vi "PH_gentec_M-Link.set Range.vi"(0 "i ref in":refnum<vi>, 2 "VISA resource in":refnum<visa-resource-name>, 5 "error in":errorcluster) -> (11 "Timeout":bool, 13 "Data read":string[](array[string]), 14 "i ref out":refnum<vi>, 16 "VISA resource out":refnum<visa-resource-name>, 17 "Error":bool, 18 "Failure":bool, 19 "error out":errorcluster)   [LabVIEW 2014, in "PH_gentec_M-Link.lvlib"]
doc: "This VI writes wanted Settings to the Device and checks the result."
uses:
  PH_gentec_M-Link.lvlib
  instr.lib/Gentec-M-Link/Driver/Type Defs/gentec-M-Link.Range Queries.ctl
  instr.lib/Gentec-M-Link/gentec-M-Link - Driver.lvlib
  PH_Basics/PH_Powermeter_BaseClass/PH_Powermeter_BaseClass.lvlib
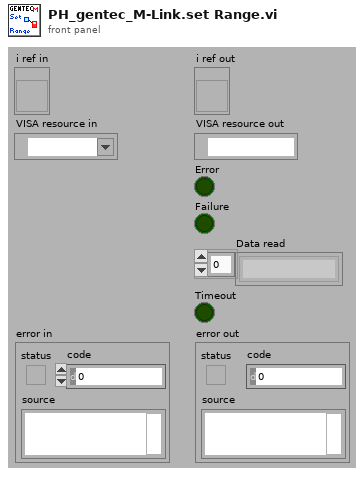
[diagram p1: front panel]
types:
  T1 = typedef "PH_Powermeter_BaseClass.lvlib/PH_Powermeter_BaseClass.i attribute.ctl" = cluster{"GUI References":T2, "Connection":T3, "Head Attributes":T5, "VISA resource":refnum<visa-resource-name>, "Energy":T6, "Service ID Energy":i32, "Wanted Settings":T7, "Current Settings":T7}
  T2 = typedef "PH_Powermeter_BaseClass.lvlib/PH_Powermeter_BaseClass.GUI Refs.ctl" = cluster{"Head Attributes":refnum<vi>, "Energy":refnum<vi>, "Connection":refnum<vi>, "VISA Resource":refnum<vi>, "Scaling Factor":refnum<vi>, "Range":refnum<vi>, "Wavelength":refnum<vi>, "Trigger Level":refnum<vi>, "Wanted Settings":refnum<vi>, "Current Settings":refnum<vi>}
  T3 = typedef "PH_Powermeter_BaseClass.lvlib/PH_Powermeter_BaseClass.Connection.ctl" = cluster{"failed checks":i8, "Timeout":bool, "Data read":string, "Failure":bool, "Error":bool, "State":T4}
  T4 = typedef "PH_Powermeter_BaseClass.lvlib/PH_Powermeter_BaseClass.State.ctl" = enum32{"off", "operating", "opened", "checked", "connected", "Sets to change", "running"}
  T5 = typedef "PH_Powermeter_BaseClass.lvlib/PH_Powermeter_BaseClass.Head Attributes.ctl" = cluster{"Instrument Type":string, "Head Version":string, "Head Name":string, "Serial Number":string, "Firmware":string, "Sensor Type":string, "MinimumRange":u32, "Maximum Range":u32, "Min Wavelength":i32, "Max Wavelength":i32}
  T6 = typedef "PH_Powermeter_BaseClass.lvlib/PH_Powermeter_BaseClass.Energy.ctl" = cluster{"current Value":dbl, "unscaled":dbl, "Scaling Factor":dbl}
  T7 = typedef "PH_Powermeter_BaseClass.lvlib/PH_gentec_BaseClass.Head Settings.ctl" = cluster{"Trigger Level":dbl, "Wavelength":u32, "Range":u32}
  T8 = typedef "gentec-M-Link - Driver.lvlib/gentec-M-Link.Range Queries.ctl" = string
  T9 = typedef "gentec-M-Link - Driver.lvlib/gentec-M-Link.Range.ctl" = u16
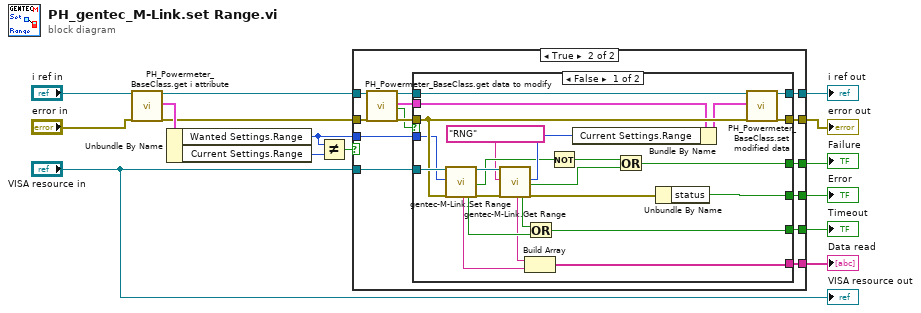
[diagram p0: block diagram]
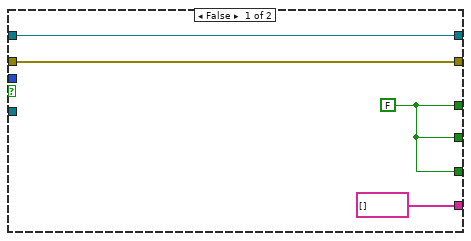
[diagram p2: hidden frame]
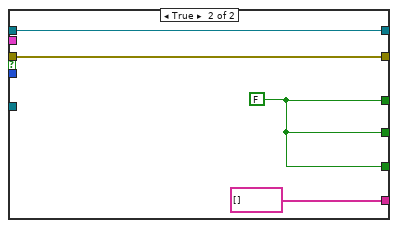
[diagram p3: hidden frame]
diagram:
  n1 = call "PH_Powermeter_BaseClass.get i attribute.vi"("i ref in"="i ref in", "error in (no error)"="error in") -> ("i ref out"=w8:refnum<vi>, "i attribute"=w11:T1, "error out"=w10:errorcluster)  [unwired: 15 in]
  n2 = Unbundle By Name(w11) -> ("Wanted Settings.Range"=w13:u32, "Current Settings.Range"=w12:u32)
  n3 = Not Equal?(x=w13, y=w12) -> (x != y?=w1:bool)
  n4 = case shown="True" w1 {
    tunnel: [w16 w33] -> w15
    tunnel: [w17 w32] -> w14
    tunnel: w13 -> [_ w31]
    tunnel: w10 -> [w16 w26]
    tunnel: w8 -> [w17 w25]
    tunnel: "VISA resource in" -> [_ w24]
    tunnel: [w19 w23] -> w5
    tunnel: [w19 w22] -> w4
    tunnel: [w19 w21] -> w3
    tunnel: [string[] [] w20] -> w2
    frame False {
      w19 = FALSE
    }
    frame True {
      n5 = call "PH_Powermeter_BaseClass.get data to modify.vi"("i ref in"=w25, "error in (no error)"=w26) -> ("i ref out"=w29:refnum<vi>, "i attribute"=w28:T1, "timed out"=w27:bool, "error out"=w30:errorcluster)  [unwired: 14 in]
      n6 = case shown="False" w27 {
        tunnel: w24 -> [w56 _]
        tunnel: [w52 w61] -> w32
        tunnel: [w51 w60] -> w33
        tunnel: w30 -> [w55 w60]
        tunnel: w29 -> [w57 w61]
        tunnel: w28 -> [w54 _]
        tunnel: w31 -> [w53 _]
        tunnel: [w49 w59] -> w23
        tunnel: [w48 w59] -> w22
        tunnel: [w47 w59] -> w21
        tunnel: [w46 string[] []] -> w20
        frame False {
          n7 = call "gentec-M-Link.Set Range.vi"("VISA resource In"=w56, "Range"=w53, "error in (no error)"=w55) -> ("Data Read"=w36:string, "Read Timeout"=w41:bool, "VISA resource Out"=w42:refnum<visa-resource-name>, "Success"=w38:bool, "error out"=w43:errorcluster)  [unwired: 12 in]
          n8 = call "gentec-M-Link.Get Range.vi"("VISA resource In"=w42, "Range Queries"=T8 "RNG", "error in (no error)"=w43) -> ("Data Read"=w35:string, "Read Timeout"=w40:bool, "Range"=w44:T9, "Error"=w39:bool, "error out"=w45:errorcluster)  [unwired: 11 in, 1 out]
          n9 = Build Array(w35, w36) -> (w46:string[])
          n10 = Or(x=w40, y=w41) -> (x .or. y?=w47:bool)
          n11 = Not(x=w38) -> (.not. x?=w37:bool)
          n12 = Bundle By Name(cluster=w54, "Current Settings.Range"=w44) -> (w50:T1)
          n13 = Or(x=w37, y=w39) -> (x .or. y?=w48:bool)
          n14 = Unbundle By Name(w45) -> ("status"=w49:bool)
          n15 = call "PH_Powermeter_BaseClass.set modified data.vi"("i ref in"=w57, "i attribute"=w50, "error in (no error)"=w55) -> ("i ref out"=w52:refnum<vi>, "error out"=w51:errorcluster)  [unwired: 15 in]
        }
        frame True {
          w59 = FALSE
        }
      }
    }
  }
  "error out" <- w15
  "i ref out" <- w14
  "Error" <- w5
  "Failure" <- w4
  "Timeout" <- w3
  "Data read" <- w2
  "VISA resource out" <- "VISA resource in"
